vi "Deconvolution.vi"(2 "Y":dbl[](array[numeric]), 3 "X * Y":dbl[](array[numeric])) -> (0 "error":i32, 1 "X":dbl[](array[numeric]))   [LabVIEW 2020, in "NI_AALPro.lvlib"]
doc: "Computes the deconvolution of the input sequences <B>X * Y</B> and <B>Y</B>."
uses:
  <vilib>/Analysis/NI_AALPro.lvlib
  <resource>/lvanlys.dll
panel:
  # "Deconvolution"
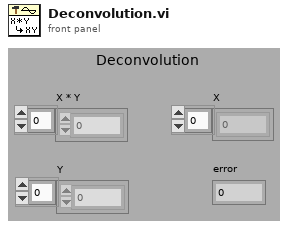
[diagram p1: front panel]
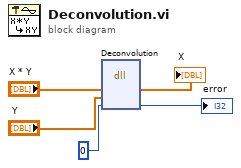
[diagram p0: block diagram]
diagram:
  n1 = dll-call lib="e:/builds/penguin/labview/branches/2020/dev/dist/resource/lvanlys.*" fn="Deconvolution"("X * Y"="X * Y", "Y"="Y", "error"=0) -> ("X * Y"=→"X":dbl[], "error"=→"error":i32)  [unwired: 5 in, 2 out]
